vi "Projectile.vi"() -> ()   [LabVIEW 2013]
uses:
  <vilib>/imath/engines/lvmath2/RunTimeEngine/ErrorHandling/NIMS_Finalize Error.vi
  <vilib>/imath/engines/lvmath2/RunTimeEngine/Managers/WorkSpace/UID Generator.vi
  <vilib>/imath/engines/lvmath2/RunTimeEngine/Managers/SymbolTable/Clear UID.vi
  <vilib>/imath/engines/lvmath2/RunTimeEngine/NodeEndStatement/NIMS_NodeEndStatement_Output.vi
  <instcachedir>/0/NIMS_NodeEndStatement_Output_53EC0D466D134D7ABD903AC30B43404B.lvgen/NIMS_NodeEndStatement_Output_53EC0D466D134D7ABD903AC30B43404B_005.vi
  <instcachedir>/0/NIMS_NodeEndStatement_Output_53EC0D466D134D7ABD903AC30B43404B.lvgen/NIMS_NodeEndStatement_Output_53EC0D466D134D7ABD903AC30B43404B_004.vi
  <vilib>/imath/engines/lvmath2/RunTimeEngine/RunTimeType/NIMS_RunTimeType_From StrictType (excl LVString).vi
  <instcachedir>/0/NIMS_RunTimeType_From StrictType (excl LVString)_57CF553C4D5778428DA95AEC531EE8B5.lvgen/NIMS_RunTimeType_From StrictType (excl LVString)_57CF553C4D5778428DA95AEC531EE8B5_000.vi
  <vilib>/imath/engines/lvmath2/RunTimeEngine/LocalVariableDefStatement/MC_LocalVariableDefStatement_Display.vi
  <vilib>/imath/engines/lvmath2/RunTimeEngine/Managers/SymbolTable/NIMS_WorkSpace.lvlib
panel:
  out "Output Cluster":T1
  out "XY Graph":cluster{"theta":i32[], "R":dbl[]}(graph)
  in  "Launch Height (m)":dbl=1.2
  in  "Launch Speed (m/s)":dbl=15.0
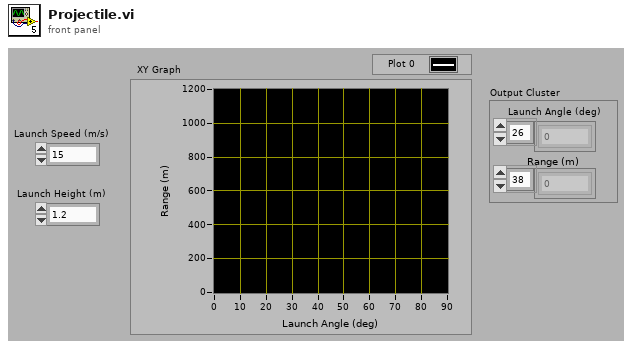
[diagram p1: front panel]
types:
  T1 = cluster{"Launch Angle (deg)":i32[], "Range (m)":dbl[]}
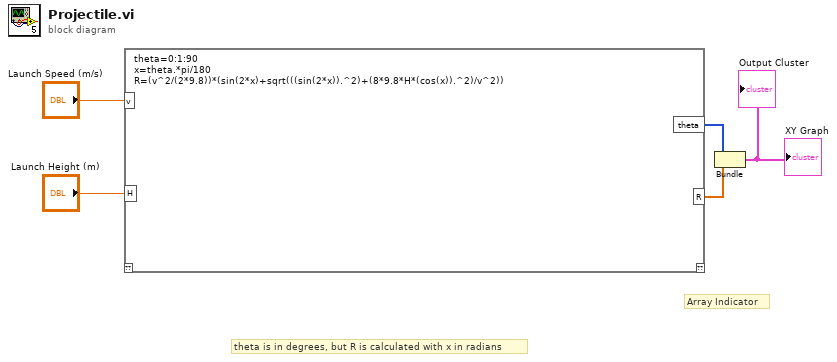
[diagram p0: block diagram]
diagram:
  # "theta is in degrees, but R is calculated with x in radians"
  # "Array Indicator"
  n1 = mathscript code="theta=0:1:90\nx=theta.*pi/180\nR=(v^2/(2*9.8))*(sin(2*x)+sqrt(((sin(2*x)).^2)+(8*9.8*H*(cos(x)).^2)/v^2))"("v"="Launch Speed (m/s)", "H"="Launch Height (m)") -> ("theta"=w5:i32[], "R"=w4:dbl[])  [unwired: 1 in, 1 out]
  n2 = Bundle("theta"=w5, "R"=w4) -> (→"XY Graph" →"Output Cluster":cluster{"theta":i32[], "R":dbl[]})  [unwired: 1 in]
